vi "Hardware - Execute Reward.vi"(8 "error in (no error)":errorcluster, 10 "Reward Time (200 ms)":u32=200) -> (0 "error out":errorcluster)   [LabVIEW 2014, in "Core SubVIs.lvlib"]
uses:
  Core SubVIs.lvlib
  <vilib>/DAQmx/write.llb/DAQmx Write (Digital Bool 1Line 1Point).vi
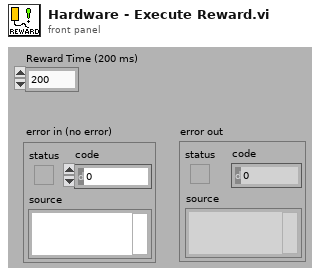
[diagram p1: front panel]
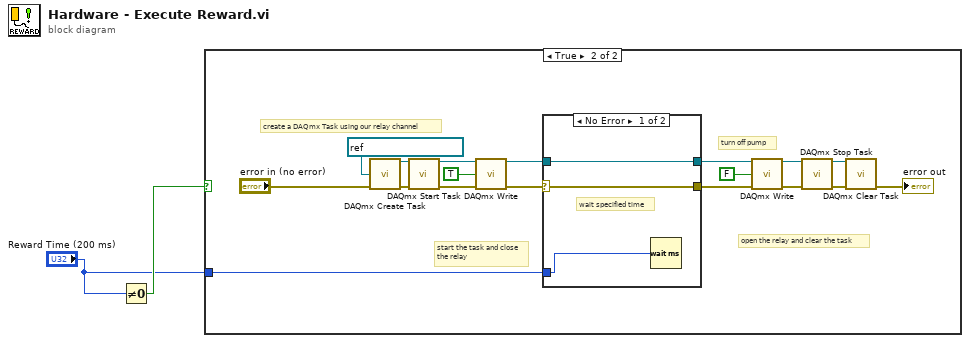
[diagram p0: block diagram]
diagram:
  n1 = Not Equal To 0?(x="Reward Time (200 ms)") -> (x != 0?=w2:bool)
  n2 = case shown="True" w2 {
    tunnel: "Reward Time (200 ms)" -> [_ w3]
    frame False {
    }
    frame True {
      # "open the relay and clear the task"
      # "start the task and close\nthe relay"
      # "create a DAQmx Task using our relay channel"
      # "turn off pump"
      n3 = call <vilib>:"DAQmx Create Task.vi"("global virtual channels"=refnum<k21> "Reward Solenoid", "error in"="error in (no error)") -> ("task out"=w19:refnum<k21>, "error out"=w18:errorcluster)  [unwired: 3 in, 9 out]
      n4 = call <vilib>:"DAQmx Start Task.vi"("task/channels in"=w19, "error in"=w18) -> ("task out"=w16:refnum<k21>, "error out"=w17:errorcluster)  [unwired: 12 out]
      n5 = call-poly <vilib>:"DAQmx Write.vi"("task/channels in"=w16, "data"=TRUE, "error in"=w17) -> ("task out"=w9:refnum<k21>, "error out"=w8:errorcluster)  [unwired: 1 in, 10 out]
      n6 = case shown="No Error" w8 {
        selector: w8 -> [w23 w24]
        tunnel: w9 -> [w22 w25]
        tunnel: [w23 w24] -> w7
        tunnel: [w22 w25] -> w6
        tunnel: w3 -> [w21 _]
        frame No Error {
          # "wait specified time"
          n7 = Wait (ms)(milliseconds to wait=w21) -> ()  [unwired: 1 out]
        }
        frame Error {
        }
      }
      n8 = call-poly <vilib>:"DAQmx Write.vi"("task/channels in"=w6, "data"=FALSE, "error in"=w7) -> ("task out"=w13:refnum<k21>, "error out"=w12:errorcluster)  [unwired: 1 in, 10 out]
      n9 = call <vilib>:"DAQmx Stop Task.vi"("task/channels in"=w13, "error in"=w12) -> ("task out"=w11:refnum<k21>, "error out"=w10:errorcluster)  [unwired: 12 out]
      n10 = call <vilib>:"DAQmx Clear Task.vi"("task in"=w11, "error in"=w10) -> ("error out"=→"error out":errorcluster)  [unwired: 13 out]
    }
  }
